vi "Th Stoch State-Space.vi"(9 "Jy":dbl=0.0038, 11 "kr":dbl=0.00064) -> (0 "Theta Deterministic State-Space Model":T1 {"Transport Delay" format="%.2f"; "D" format="%#.2g"; "C" format="%#.2g"; "B" format="%#.2g"; "A" format="%#.2g"; "properties"."Sampling Time" format="%#.6p"; "properties"."Output Delays" format="%.4f"; "properties"."Input Delays" format="%.4f"}, 1 "Theta Stochastic State-Space Model":T3 {"H" format="%#.2g"; "D" format="%#.2g"; "C" format="%#.2g"; "A" format="%#.2g"; "B" format="%#.2g"; "G" format="%#.2g"; "Sampling Time (s)" format="%.2f"}, 3 "Equation":picture, 4 "Controllability Matrix":dbl[][](array[numeric])=[[1.0, 0.0, 6.0], [0.0, 1.0, -1.0], [0.0, 0.0, 0.0]] format="%.2f", 5 "Is Controllable":bool, 6 "Observability  Matrix":dbl[][](array[numeric]) format="%#.2g", 7 "Is Observable":bool)   [LabVIEW 2017]
uses:
  <vilib>/addons/Control Design/_Stochastic Systems/Stochastic Systems.llb/Stochastic Systems SubVIs/cd_Stochastic State-Space Model.ctl
  <vilib>/addons/Control Design/_Model Construction/Model Typedefs.llb/CD State Space Model (MIMO).ctl
  <vilib>/addons/Control Design/_Model Construction/Model Typedefs.llb/CD General Elements.ctl
  <vilib>/Analysis/7linalg.llb/Create Special Real Matrix.vi
  <vilib>/addons/Control Design/_Stochastic Systems/Stochastic Systems.llb/CD Construct Stochastic Model (Numeric).vi
  <vilib>/addons/Control Design/_Stochastic Systems/NI_CD_Stochastic Systems.lvlib
  <vilib>/Analysis/NI_AALPro.lvlib
  <vilib>/addons/Control Design/_Utility/NI_CD_Model Viewer.lvlib
  <vilib>/addons/Control Design/_State-Space Analysis/NI_CD_State-Space Analysis.lvlib
  <vilib>/addons/Control Design/_Model Construction/NI_LinSys_Model Typedefs.lvlib
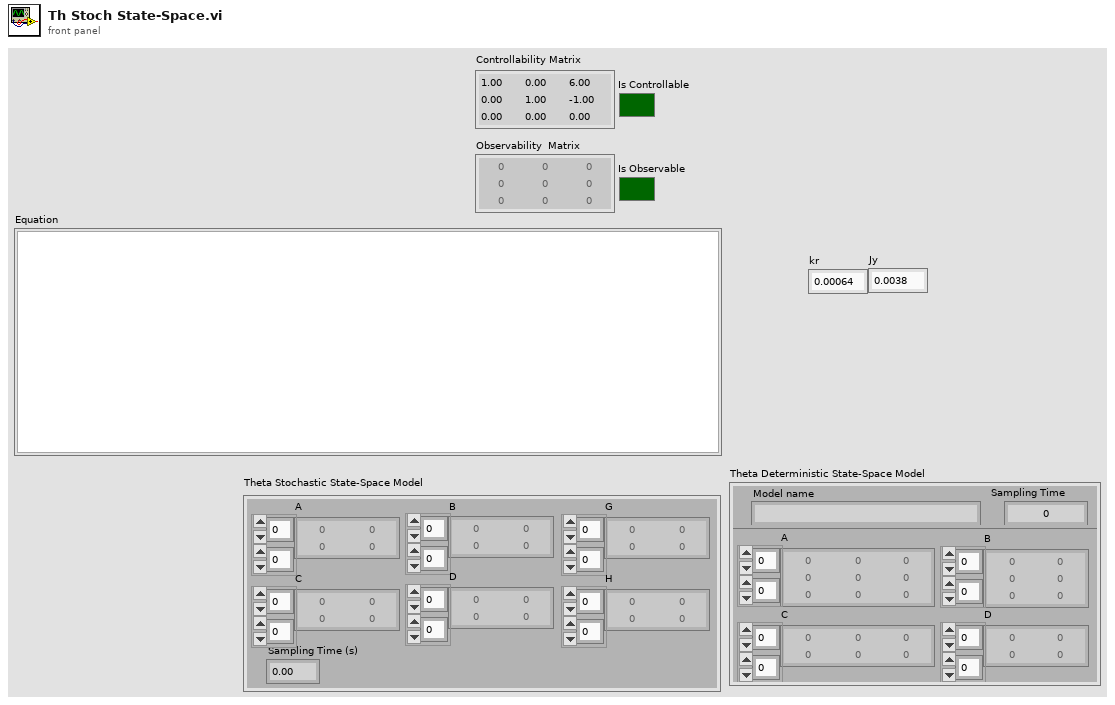
[diagram p1: front panel]
types:
  T1 = typedef "NI_LinSys_Model Typedefs.lvlib/CD State Space Model (MIMO).ctl" = cluster{"properties":T2, "A":dbl[][], "B":dbl[][], "C":dbl[][], "D":dbl[][], "StateNames":string[], "Transport Delay":dbl[][]}
  T2 = typedef "NI_LinSys_Model Typedefs.lvlib/CD General Elements.ctl" = cluster{"Model name":string, "Input names":string[], "Output names":string[], "Input Delays":dbl[], "Output Delays":dbl[], "Sampling Time":dbl, "Notes":string}
  T3 = typedef "NI_CD_Stochastic Systems.lvlib/cd_Stochastic State-Space Model.ctl" = cluster{"Sampling Time (s)":dbl, "G":dbl[][], "B":dbl[][], "A":dbl[][], "C":dbl[][], "D":dbl[][], "H":dbl[][]}
  T4 = typedef "NI_Matrix.lvlib/RealMatrix.ctl" = dbl[][]
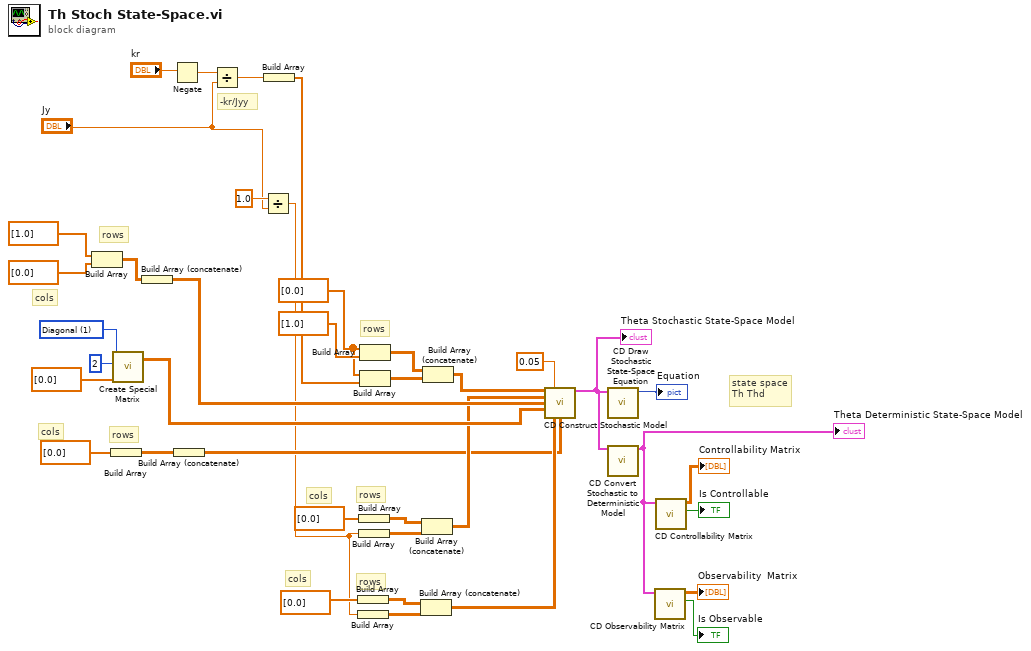
[diagram p0: block diagram]
diagram:
  w36 = 1 items=["Identity", "Diagonal", "Toepliz", "Vandermonde", "Companion", "Hankel", "Hadamard", "Wilkinson", "Hilbert", "Inverse Hilbert", "Rosser", "Pascal"] ("matrix type")
  w18 = dbl[] [0.0] ("element")
  # "-kr/Jyy"
  # "state space\nTh Thd"
  # "rows"
  # "cols"
  # "rows"
  # "cols"
  # "rows"
  # "cols"
  # "rows"
  # "cols"
  # "rows"
  n1 = Build Array(dbl[] [1.0] ("element"), dbl[] [0.0] ("element")) -> (w34:T4)
  n2 = Build Array(dbl[] [0.0] ("element")) -> (w10:T4)
  n3 = call-poly <vilib>:"Create Special Matrix.vi"("matrix type"=w36, "matrix size"=2, "Input Vector1"=dbl[] [0.0]) -> ("Special Matrix"=w31:T4)  [unwired: 2 in, 1 out]
  n4 = Build Array (concatenate)(w34) -> (w32:T4)
  n5 = Negate(x="kr") -> (-x=w6:dbl)
  n6 = Build Array (concatenate)(w10) -> (w9:T4)
  n7 = Divide(x=w6, y="Jy") -> (x/y=w5:dbl)
  n8 = Divide(x=1.0 ("ut"), y="Jy") -> (x/y=w3:dbl)
  n9 = Build Array(w5) -> (w4:dbl[])
  n10 = Build Array(dbl[] [0.0] ("element")) -> (w14:T4)
  n11 = Build Array(w3) -> (w13:T4)
  n12 = Build Array(dbl[] [0.0] ("element")) -> (w37:T4)
  n13 = Build Array(w3) -> (w15:T4)
  n14 = Build Array(w18, dbl[] [1.0] ("element")) -> (w38:T4)
  n15 = Build Array(w18, w4) -> (w39:T4)
  n16 = Build Array (concatenate)(w14, w13) -> (w12:T4)
  n17 = Build Array (concatenate)(w37, w15) -> (w28:T4)
  n18 = Build Array (concatenate)(w38, w39) -> (w33:T4)
  n19 = call-poly <vilib>:"CD Construct Stochastic Model.vi"("A"=w33, "Sampling Time (s)"=0.05, "B"=w28, "C"=w32, "D"=w31, "G"=w12, "H"=w9) -> ("Stochastic State-Space Model"=w26:T3)  [unwired: 7 in, 1 out]
  "Theta Stochastic State-Space Model" <- w26
  n20 = call <vilib>:"CD Draw Stochastic State-Space Equation.vi"("Stochastic State-Space Model"=w26) -> ("Equation"=→"Equation":picture)  [unwired: 8 in, 2 out]
  n21 = call <vilib>:"CD Convert Stochastic to Deterministic Model.vi"("Stochastic State-Space Model"=w26) -> ("Deterministic State-Space Model"=w24:T1)  [unwired: 13 in, 1 out]
  "Theta Deterministic State-Space Model" <- w24
  n22 = call <vilib>:"CD Observability Matrix.vi"("State-Space Model"=w24) -> ("Is Observable?"=→"Is Observable":bool, "Observability  Matrix"=→"Observability  Matrix":dbl[][])  [unwired: 7 in, 2 out]
  n23 = call <vilib>:"CD Controllability Matrix.vi"("State-Space Model"=w24) -> ("Is Controllable?"=→"Is Controllable":bool, "Controllability Matrix"=→"Controllability Matrix":dbl[][])  [unwired: 7 in, 2 out]
